vi "Program list Selection.vi"(8 "error in":errorcluster, 9 "FeedBack Channel":string[](array[string])=["fgdgfvcbc", "vnfhgjkn", "21354682"], 10 "Filepath":path=path "D:/My Project/2019-2020/Magnetic Mareli UM/MM_UM/Project Setup/data/program seq/Program_280A.bin", 11 "vi referenceIn":refnum<vi>) -> (0 "error out":errorcluster, 1 "Exit":bool, 2 "String":string, 3 "vi reference Out":refnum<vi>)   [LabVIEW 2015]
uses:
  Control Button/Exit.ctl
  Control Button/next.ctl
  Galobal variable_TI.vi
  <vilib>/addons/database/Connection.llb/DB Tools Open Connec (String).vi
  <vilib>/addons/database/_DB Variant To Data/Database Variant To Data.xnode
  <vilib>/addons/database/NI_Database_API.lvlib
panel:
  in  "Setting Data":T1
  out "error out 2":errorcluster
  out "data":T1
  out "String 2":string
  in  "Next":T2
  in  "Exit":T3
  in  "Program List":string(combo)
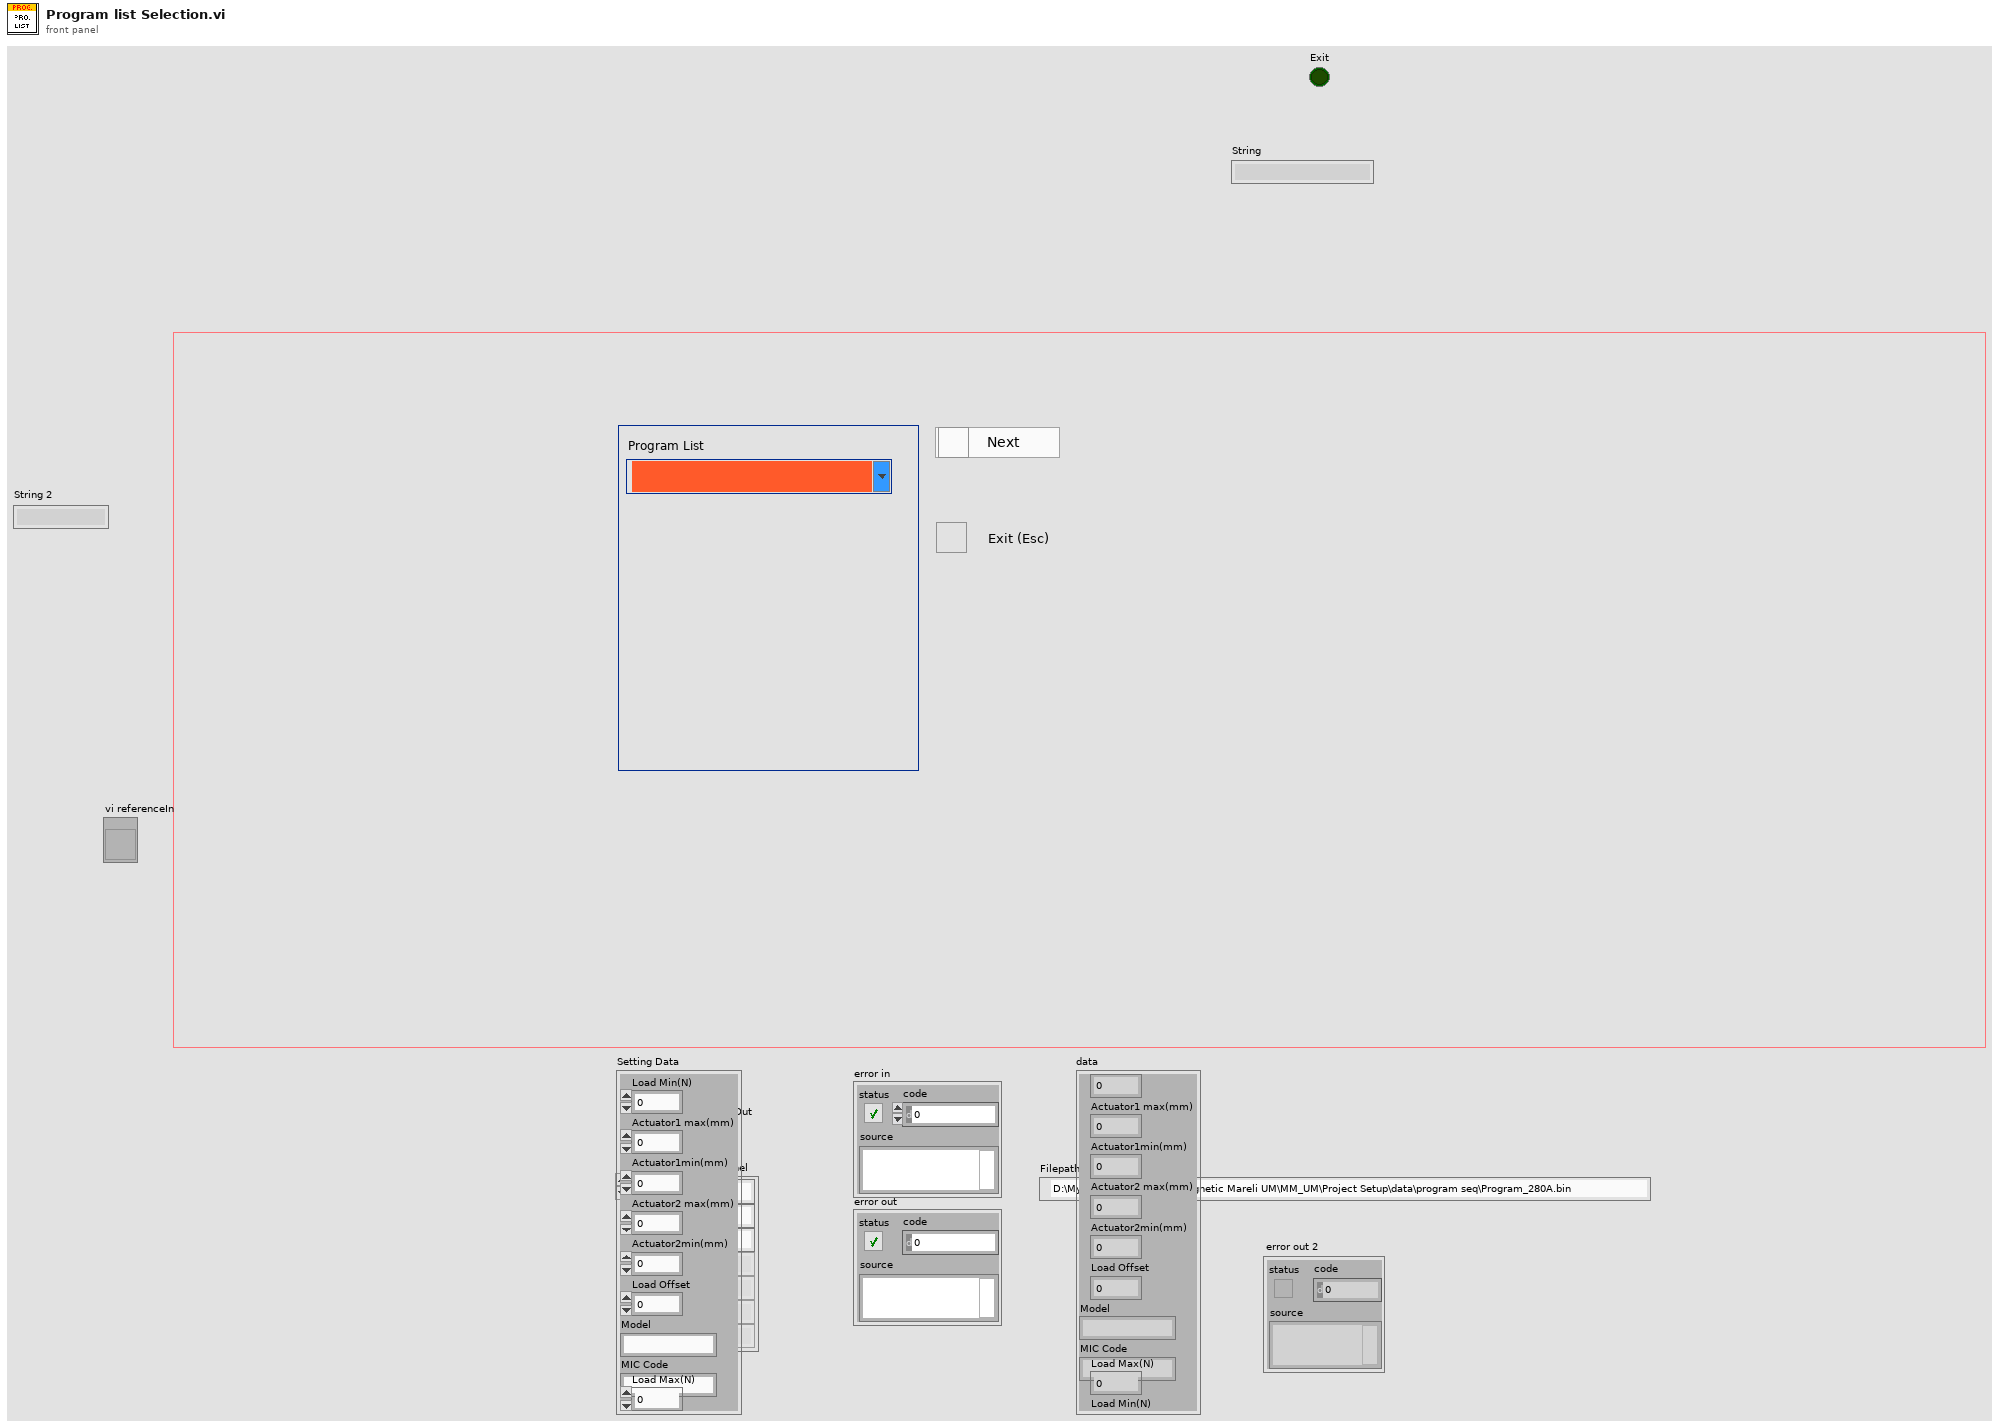
[diagram p1: front panel]
types:
  T1 = cluster{"Load Max(N)":dbl, "Load Min(N)":dbl, "Actuator1 max(mm)":dbl, "Actuator1min(mm)":dbl, "Actuator2 max(mm)":dbl, "Actuator2min(mm)":dbl, "Load Offset":dbl, "Model":string, "MIC Code":string}
  T2 = typedef "next.ctl" = bool
  T3 = typedef "Exit.ctl" = bool
  T4 = enum32{"Invalid", "Standard", "Closed", "Hidden", "Minimized", "Maximized"}
  T5 = typedef "NI_Database_API.lvlib/Conn ObjectReference.ctl" = refnum<k1>
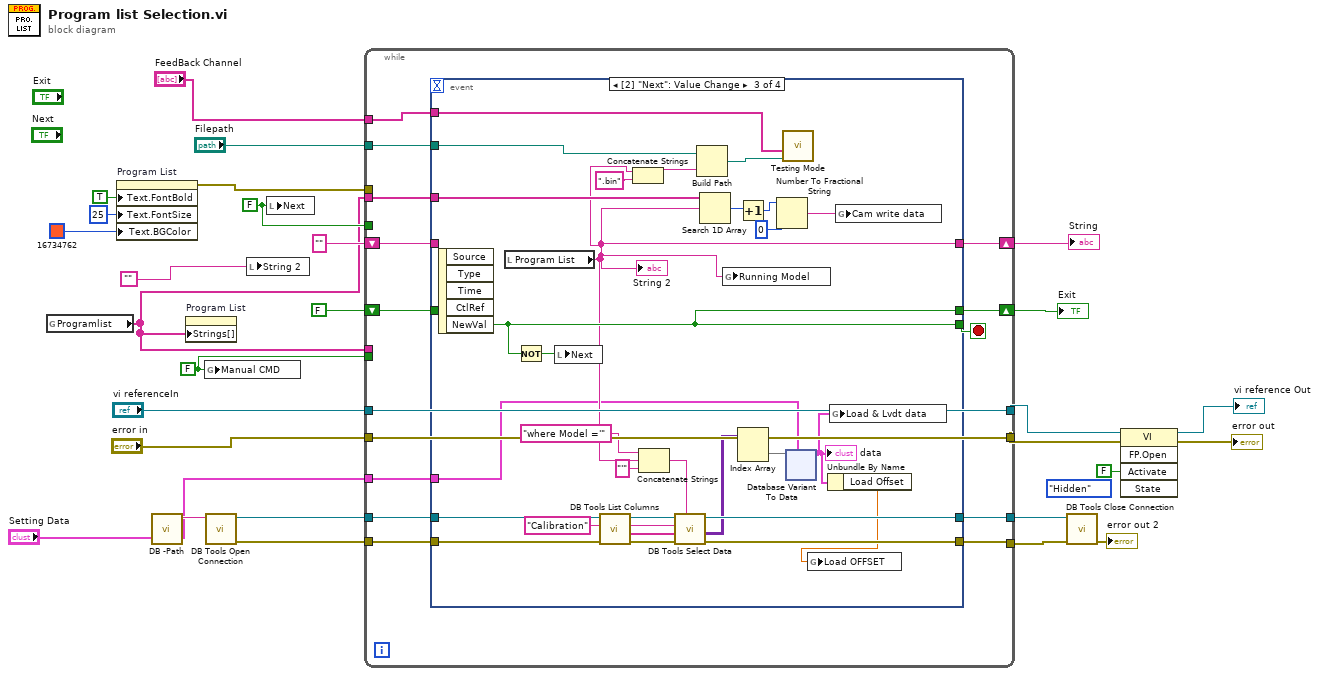
[diagram p0: block diagram]
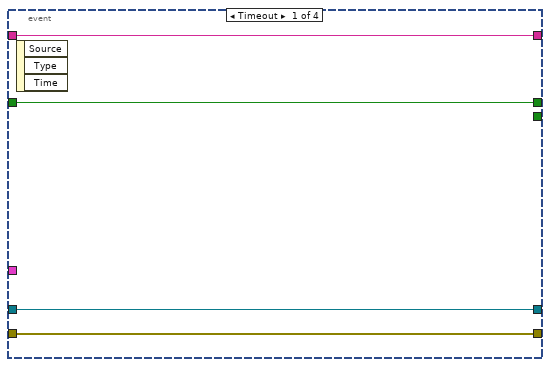
[diagram p2: hidden frame]
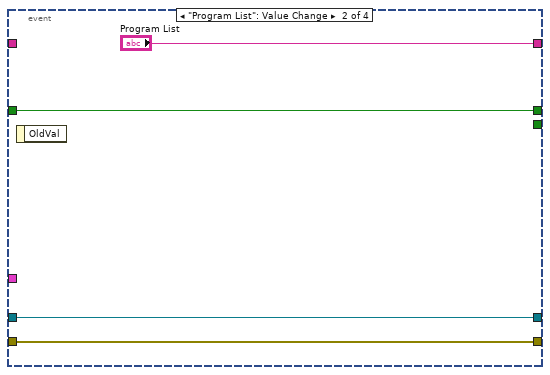
[diagram p3: hidden frame]
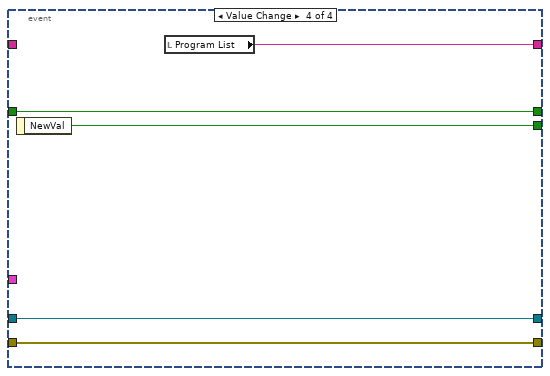
[diagram p4: hidden frame]
diagram:
  (unwired) T4."Hidden" ("State")
  w18 = FALSE ("Manual CMD")
  w19 = FALSE ("Next")
  n1 = global read "Galobal variable_TI.vi" "Programlist"() -> (w8:string[])
  n2 = property on="Program List" class="CmbBox"("Text.FontBold"=TRUE ("Text.Font:Bold"), "Text.FontSize"=u32 25 ("Text.Font:Size"), "Text.BGColor"=u32 16734762 ("Color Box")) -> (error out=w22:errorcluster)  [unwired: 2 in, 1 out]
  n3 = call "DB -Path.vi"() -> ("String"=w7:string)  [unwired: 11 in]
  n4 = property on="Program List" class="CmbBox"("Strings[]"=w8) -> ()  [unwired: 2 in, 2 out]
  n5 = global write "Galobal variable_TI.vi" "Manual CMD"(w18) -> ()
  n6 = call-poly <vilib>:"DB Tools Open Connection.vi"("connection information"=w7) -> ("error out"=w5:errorcluster, "connection reference"=w6:T5)  [unwired: 7 in]
  n7 = local write "String 2"("") -> ()
  n8 = local write "Next"(w19) -> ()
  n9 = while {
    shift-right: [w43] -> w28
    shift-left: "" ("Combo Box") -> [w42]
    shift-right: [w40] -> w25
    shift-left: T3 FALSE ("NewVal") -> [w39]
    tunnel: w8 -> [_]
    tunnel: w22 -> [_]
    tunnel: w19 -> [_]
    tunnel: w18 -> [_]
    tunnel: "vi referenceIn" -> [w38]
    tunnel: [w38] -> w12
    tunnel: "error in" -> [w37]
    tunnel: [w37] -> w11
    tunnel: "Filepath" -> [w36]
    tunnel: "FeedBack Channel" -> [w35]
    tunnel: w8 -> [w34]
    tunnel: w6 -> [w33]
    tunnel: w5 -> [w32]
    tunnel: [w31] -> w3
    tunnel: [w30] -> w2
    tunnel: "Setting Data" -> [w29]
    stop <- w41 stop-if-true
    n10 = event shown="[2] \"Next\": Value Change" {
      selector: _ -> [_ _ _ _]
      dyn-events: _ -> [_ _ _ _]
      timeout: _ -> [_ _ _ _]
      tunnel: [w47 "Program List" w59 w367] -> w43
      tunnel: w42 -> [w47 _ _ _]
      tunnel: [_ _ w75 w368] -> w41
      tunnel: [w46 w50 w75 w366] -> w40
      tunnel: w39 -> [w46 w50 _ w366]
      tunnel: w36 -> [_ _ w78 _]
      tunnel: w35 -> [_ _ w76 _]
      tunnel: w34 -> [_ _ w73 _]
      tunnel: w33 -> [w44 w48 w63 w364]
      tunnel: w32 -> [w45 w49 w62 w365]
      tunnel: [w44 w48 w61 w364] -> w31
      tunnel: [w45 w49 w60 w365] -> w30
      tunnel: w29 -> [_ _ w56 _]
      event Timeout {
        n11 = event-data() -> ()  [unwired: 1 in, 3 out]
      }
      event "Program List": Value Change {
        n12 = event-data() -> ()  [unwired: 1 in, 1 out]
      }
      event Value Change {
        w64 = "Calibration" ("table")
        n13 = event-data() -> ("NewVal"=w75:T2)  [unwired: 1 in, 4 out]
        n14 = local read "Program List"() -> (w59:string)
        "String 2" <- w59
        n15 = Not(x=w75) -> (.not. x?=w74:T2)
        n16 = local write "Next"(w74) -> ()
        n17 = call <vilib>:"DB Tools List Columns.vi"("error in (no error)"=w62, "table"=w64, "connection reference"=w63) -> ("error out"=w70:errorcluster, "columns"=w68:string[], "connection reference out"=w69:T5)  [unwired: 1 in, 1 out]
        n18 = Concatenate Strings(w59, ".bin" ("string")) -> (w79:string)
        n19 = Concatenate Strings("where Model ='" ("string"), w59, "'" ("string")) -> (w65:string)
        n20 = call <vilib>:"DB Tools Select Data.vi"("condition"=w65, "error in (no error)"=w70, "columns"=w68, "table"=w64, "connection reference"=w69) -> ("error out"=w60:errorcluster, "data"=w58:variant[][], "connection reference out"=w61:T5)  [unwired: 1 in]
        n21 = Build Path(base path=w78, name or relative path=w79) -> (appended path=w77:path)
        n22 = Search 1D Array(1D array=w73, element=w59) -> (index of element=w72:i32)  [unwired: 1 in]
        n23 = global write "Galobal variable_TI.vi" "Running Model"(w59) -> ()
        n24 = Increment(x=w72) -> (x+1=w71:i32)
        n25 = Index Array(array=w58) -> (element=w57:variant[])  [unwired: 2 in]
        n26 = Number To Fractional String(number=w71, precision (6)=i16 0) -> (F-format string=w53:string)  [unwired: 2 in]
        n27 = call "Testing Mode.vi"("Filepath"=w77, "FeedBack Channel"=w76) -> ()  [unwired: 10 in]
        n28 = xnode "Database Variant To Data"("database variant"=w57, "type"=w56) -> ("data"=w55:T1)  [unwired: 1 in, 1 out]
        "data" <- w55
        n29 = Unbundle By Name(w55) -> ("Load Offset"=w54:dbl)
        n30 = global write "Galobal variable_TI.vi" "Load OFFSET"(w54) -> ()
        n31 = global write "Galobal variable_TI.vi" "Load & Lvdt data"(w55) -> ()
        n32 = global write "Galobal variable_TI.vi" "Cam write data"(w53) -> ()
      }
      event Value Change {
        n33 = event-data() -> ("NewVal"=w368:T3)  [unwired: 1 in]
        n34 = local read "Program List"() -> (w367:string)
      }
    }
  }
  "String" <- w28
  "Exit" <- w25
  n35 = call <vilib>:"DB Tools Close Connection.vi"("error in (no error)"=w2, "connection reference"=w3) -> ("error out"=→"error out 2":errorcluster)  [unwired: 5 in]
  n36 = invoke class="VI" method="FP.Open"(reference=w12, error in=w11, "Activate"=FALSE ("Activate?")) -> (reference out=→"vi reference Out":refnum<vi>, error out=→"error out":errorcluster)  [unwired: 2 in, 3 out]
